vi "Main.vi"(8 "error in":errorcluster, 11 "GraphShow in":refnum<class "GraphShow.lvclass">) -> (0 "error out":errorcluster, 3 "GraphShow out":refnum<class "GraphShow.lvclass">)   [LabVIEW 2024, in "GraphShow.lvclass"]
doc: "The <b>Queued Message Handler</b> of the Worker that owns this VI."
uses:
  GraphShow.lvclass
  C:/Program Files (x86)/National Instruments/LabVIEW 2024/vi.lib/addons/_Workers/Library/Classes/Worker/Worker.lvclass
  Initialization Data.ctl
  Response Cases.ctl
  GraphShow.lvclass/GraphShow.ctl
  rql_RandomPattern.ctl
  rql_PanelDataUpdate.ctl
  <vilib>/addons/_Workers/Library/Classes/Message Queue/Message Queue.lvclass
  <vilib>/Analysis/NI_AALBase.lvlib
  e282c702-d748-4358-84ac-45f283b9f1c7.vi
panel:
  out "XY Graph":cluster{"sine wave":dbl[], "sine wave":dbl[]}(graph)
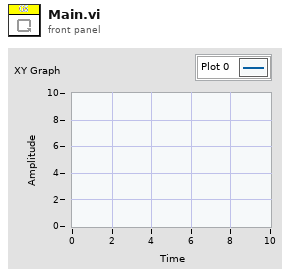
[diagram p1: front panel]
types:
  T1 = typedef "GraphShow.lvclass/Initialization Data.ctl" = cluster{"Response Cases":T2}
  T2 = typedef "GraphShow.lvclass/Response Cases.ctl" = cluster{"Placeholder - Can be deleted":string}
  T3 = typedef "GraphShow.lvclass/rql_RandomPattern.ctl" = cluster{"String":string}
  T4 = typedef "GraphShow.lvclass/rql_PanelDataUpdate.ctl" = cluster{"String":string}
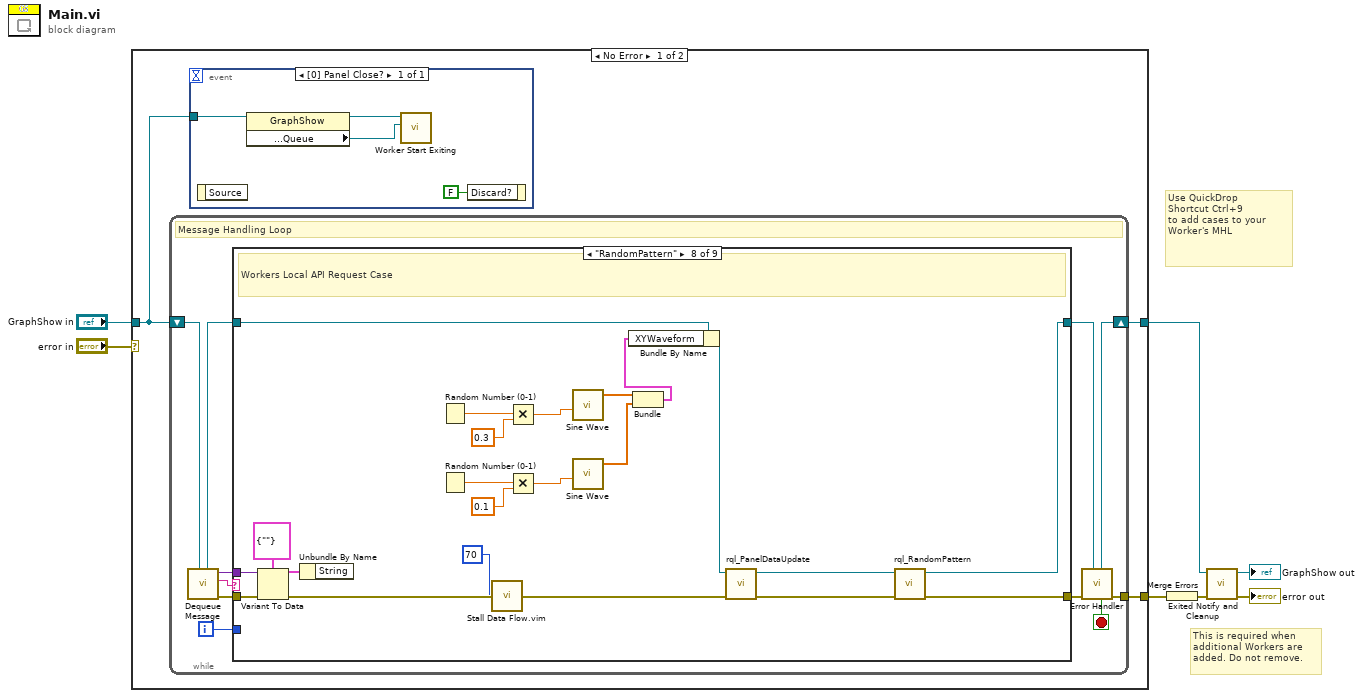
[diagram p0: block diagram]
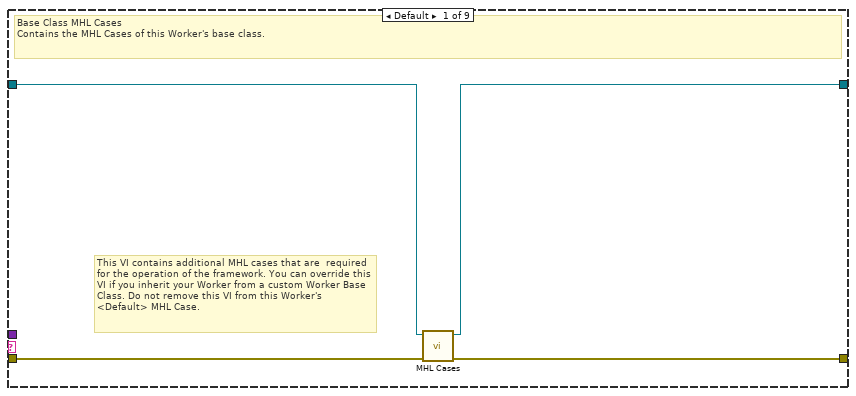
[diagram p2: hidden frame]
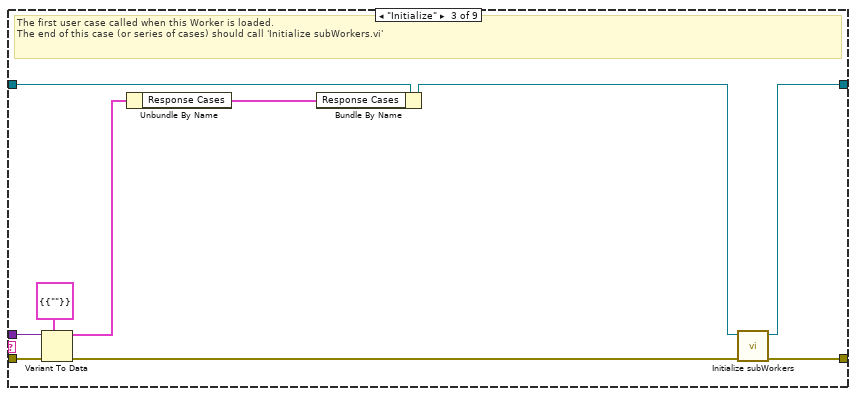
[diagram p4: hidden frame]
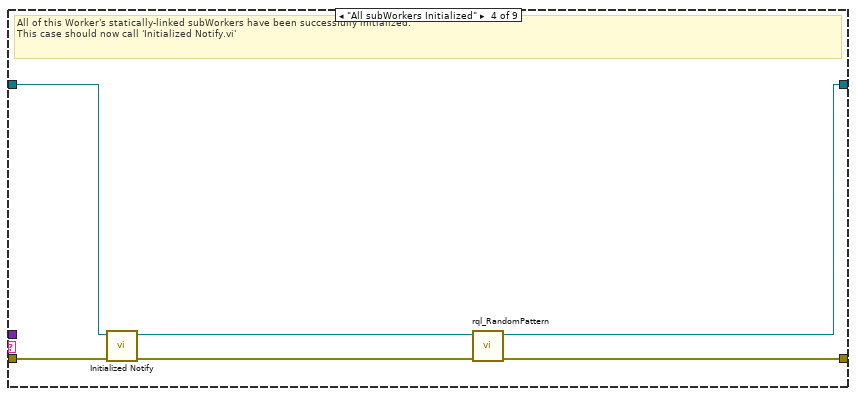
[diagram p5: hidden frame]
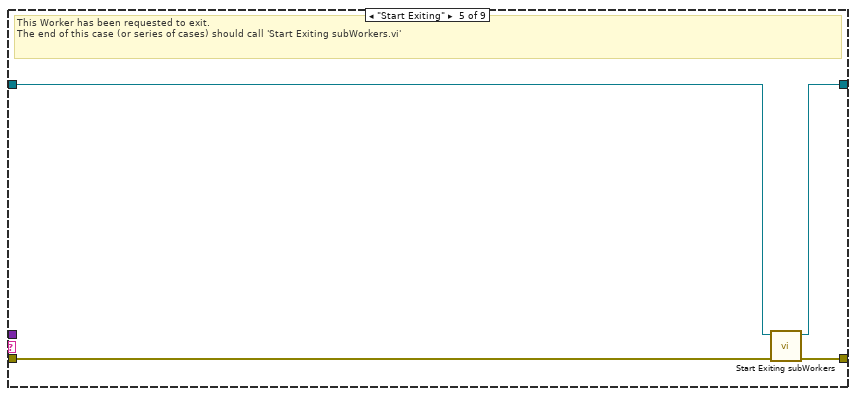
[diagram p6: hidden frame]
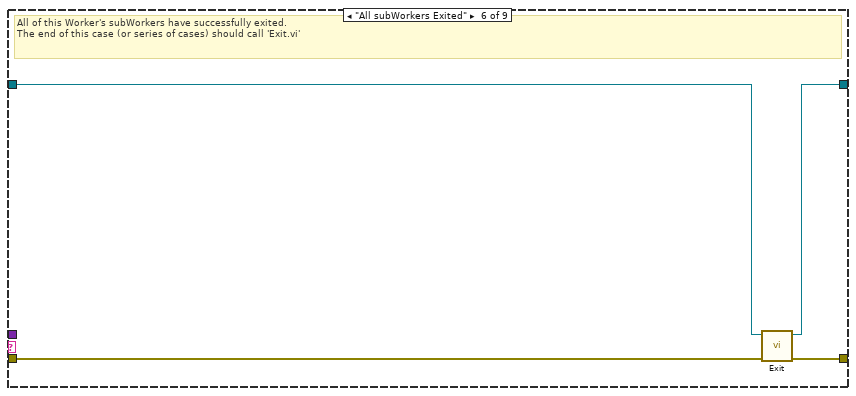
[diagram p7: hidden frame]
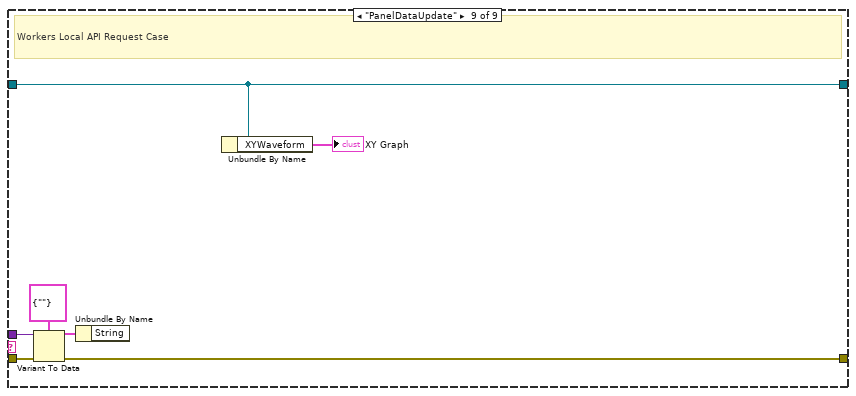
[diagram p9: hidden frame]
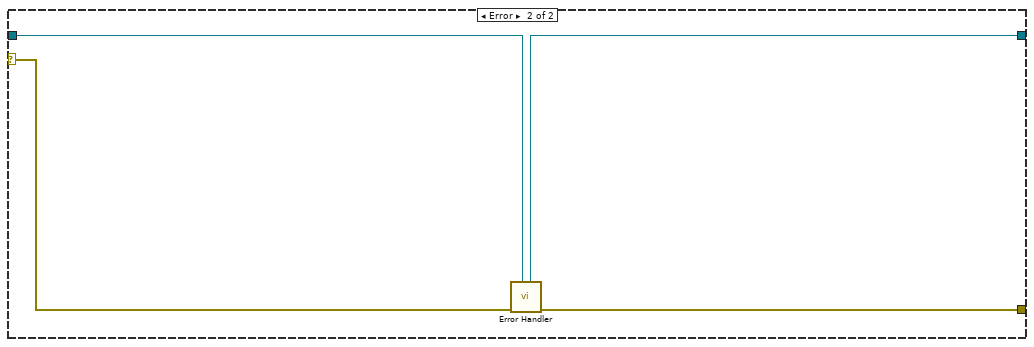
[diagram p10: hidden frame]
diagram:
  # "Use QuickDrop\nShortcut Ctrl+9\nto add cases to your\nWorker's MHL"
  # "This is required when additional Workers are added. Do not remove."
  n1 = case shown="No Error" "error in" {
    tunnel: "GraphShow in" -> [w8 w88]
    tunnel: [w10 w89] -> w6
    tunnel: [w9 w87] -> w7
    selector: "error in" -> [_ w90]
    frame No Error {
      n2 = while {
        shift-right: [w23] -> w9
        shift-left: w8 -> [w25]
        tunnel: [w24] -> w10
        i -> [w16]
        stop <- w17 stop-if-true
        # "Message Handling Loop"
        n3 = call-dynamic "Dequeue Message.vi"("Worker"=w25) -> ("error out"=w22:errorcluster, "Case out"=w18:string, "Data out"=w15:variant, "Worker out"=w20:refnum<class "GraphShow.lvclass">)  [unwired: 6 in, 1 out]
        n4 = case "Worker MHL Case Structure (DO NOT CHANGE LABEL NAME)" shown="\"RandomPattern\"" w18 {
          tunnel: w22 -> [w29 w30 w39 w47 w48 w55 w57 w78 w86]
          tunnel: [w28 w30 w41 w44 w51 w54 w57 w62 w85] -> w21
          tunnel: w20 -> [w27 w31 w38 w45 w49 w53 w56 w79 w81]
          tunnel: [w26 w31 w40 w42 w50 w52 w56 w60 w81] -> w19
          tunnel: w16 -> [_ _ _ _ _ _ _ _ _]
          tunnel: w15 -> [_ _ w36 _ _ _ _ w75 w83]
          frame Default {
            # "This VI contains additional MHL cases that are  required for the operation of the framework. You can override this VI if you inherit your Worker from a custom Worker Base Class. Do not remove this VI from this Worker's <Default> MHL Case."
            # "Base Class MHL Cases\nContains the MHL Cases of this Worker's base class."
            n5 = call-dynamic "MHL Cases.vi"("error in"=w29, "Worker in"=w27) -> ("error out"=w28:errorcluster, "Worker out"=w26:refnum<class "GraphShow.lvclass">)  [unwired: 8 in]
          }
          frame "------------ FRAMEWORK CASES -----------" {
            # "Start of Workers Framework Cases"
          }
          frame "Initialize" {
            # "The first user case called when this Worker is loaded.\nThe end of this case (or series of cases) should call 'Initialize subWorkers.vi'"
            n6 = Variant To Data(error in=w39, type=T1 {"Response Cases"={"Placeholder - Can be deleted"=""}} ("Cluster"), Variant=w36) -> (data=w34:T1, error out=w37:errorcluster)
            n7 = Unbundle By Name(w34) -> ("Response Cases"=w33:T2)
            n8 = Bundle By Name(cluster=w38, "Response Cases"=w33) -> (w35:refnum<class "GraphShow.lvclass">)
            n9 = call-dynamic "Initialize subWorkers.vi"("error in"=w37, "Worker"=w35) -> ("error out"=w41:errorcluster, "dup Worker out"=w40:refnum<class "GraphShow.lvclass">)  [unwired: 8 in]
          }
          frame "All subWorkers Initialized" {
            # "All of this Worker's statically-linked subWorkers have been successfully initialized.\nThis case should now call 'Initialized Notify.vi'"
            n10 = call-dynamic "Initialized Notify.vi"("error in"=w47, "Worker"=w45) -> ("error out"=w46:errorcluster, "dup Worker out"=w43:refnum<class "GraphShow.lvclass">)  [unwired: 8 in]
            n11 = call "rql_RandomPattern.vi"("error in"=w46, "GraphShow in"=w43) -> ("error out"=w44:errorcluster, "dup GraphShow out"=w42:refnum<class "GraphShow.lvclass">)  [unwired: 8 in]
          }
          frame "Start Exiting" {
            # "This Worker has been requested to exit. \nThe end of this case (or series of cases) should call 'Start Exiting subWorkers.vi'"
            n12 = call-dynamic "Start Exiting subWorkers.vi"("error_in"=w48, "Worker"=w49) -> ("error out"=w51:errorcluster, "dup Worker out"=w50:refnum<class "GraphShow.lvclass">)  [unwired: 8 in]
          }
          frame "All subWorkers Exited" {
            # "All of this Worker's subWorkers have successfully exited. \nThe end of this case (or series of cases) should call 'Exit.vi'"
            n13 = call-dynamic "Exit.vi"("error_in"=w55, "Worker"=w53) -> ("error out"=w54:errorcluster, "dup Worker out"=w52:refnum<class "GraphShow.lvclass">)  [unwired: 8 in]
          }
          frame "------------- LOCAL API CASES -------------" {
            # "Start of Workers Local API Cases"
          }
          frame "RandomPattern" {
            # "Workers Local API Request Case"
            n14 = Variant To Data(error in=w78, type=T3 {"String"=""} ("Data"), Variant=w75) -> (data=w74:T3, error out=w77:errorcluster)
            n15 = Unbundle By Name(w74) -> ()  [unwired: 1 out]
            n16 = Random Number (0-1)() -> (number: 0 to 1=w73:dbl)
            n17 = Random Number (0-1)() -> (number: 0 to 1=w68:dbl)
            n18 = call "Stall Data Flow.vim"("value in"=w77, "milliseconds to wait"=u32 70) -> ("value out"=w59:errorcluster)  [unwired: 1 out]
            n19 = Multiply(x=w73, y=0.3) -> (x*y=w72:dbl)
            n20 = Multiply(x=w68, y=0.1) -> (x*y=w69:dbl)
            n21 = call <vilib>:"Sine Wave.vi"("frequency"=w72) -> ("sine wave"=w67:dbl[])  [unwired: 4 in, 2 out]
            n22 = call <vilib>:"Sine Wave.vi"("frequency"=w69) -> ("sine wave"=w66:dbl[])  [unwired: 4 in, 2 out]
            n23 = Bundle("sine wave"=w67, "sine wave"=w66) -> (w65:cluster{"sine wave":dbl[], "sine wave":dbl[]})  [unwired: 1 in]
            n24 = Bundle By Name(cluster=w79, "XYWaveform"=w65) -> (w64:refnum<class "GraphShow.lvclass">)
            n25 = call "rql_PanelDataUpdate.vi"("error in"=w59, "GraphShow in"=w64) -> ("error out"=w63:errorcluster, "dup GraphShow out"=w61:refnum<class "GraphShow.lvclass">)  [unwired: 8 in]
            n26 = call "rql_RandomPattern.vi"("error in"=w63, "GraphShow in"=w61) -> ("error out"=w62:errorcluster, "dup GraphShow out"=w60:refnum<class "GraphShow.lvclass">)  [unwired: 8 in]
          }
          frame "PanelDataUpdate" {
            # "Workers Local API Request Case"
            n27 = Variant To Data(error in=w86, type=T4 {"String"=""} ("Data"), Variant=w83) -> (data=w82:T4, error out=w85:errorcluster)
            n28 = Unbundle By Name(w82) -> ()  [unwired: 1 out]
            n29 = Unbundle By Name(w81) -> ("XYWaveform"=→"XY Graph":cluster{"sine wave":dbl[], "sine wave":dbl[]})
          }
        }
        n30 = call-dynamic "Error Handler.vi"("Worker"=w19, "error_in"=w21) -> ("error out"=w24:errorcluster, "Stop Loop"=w17:bool, "Worker out"=w23:refnum<class "GraphShow.lvclass">)  [unwired: 7 in]
      }
      n31 = event shown="[0] Panel Close?" {
        selector: _ -> [_]
        dyn-events: _ -> [_]
        timeout: _ -> [_]
        tunnel: w8 -> [w13]
        event Panel Close? {
          n32 = event-data() -> ()  [unwired: 1 in, 1 out]
          n33 = property class="GraphShow"(reference=w13) -> (reference out=w12:refnum<class "GraphShow.lvclass">, "Accessors:Read:Public API:Queue"=w11:refnum<class "Message Queue.lvclass">)  [unwired: 1 in, 1 out]
          n34 = call-dynamic "Worker Start Exiting.vi"("Message Queue"=w11, "Worker"=w12) -> ()  [unwired: 8 in, 2 out]
          n35 = event-data("Discard?"=FALSE) -> ()  [unwired: 1 in, 1 out]
        }
      }
    }
    frame Error {
      n36 = call-dynamic "Error Handler.vi"("Worker"=w88, "error_in"=w90) -> ("error out"=w89:errorcluster, "Worker out"=w87:refnum<class "GraphShow.lvclass">)  [unwired: 7 in, 1 out]
    }
  }
  n37 = Merge Errors(w6) -> (w3:errorcluster)
  n38 = call-dynamic "Exited Notify and Cleanup.vi"("error_in"=w3, "Worker"=w7) -> ("error out"=→"error out":errorcluster, "dup Worker out"=→"GraphShow out":refnum<class "GraphShow.lvclass">)  [unwired: 8 in]
